vi "MOV_Query.vi"(0 "System no.":i32=1 min=1 max=4 step=1, 2 "Axes to query":string[](array[string]), 3 "All axes?":bool, 4 "Axis identifier?":bool=TRUE, 5 "error in":errorcluster) -> (14 "Target position":dbl[](array[numeric]) format="%.6f", 19 "error out":errorcluster)   [LabVIEW 2020]
doc: "GCS 3.0\n=====\n\nMOV? (Get Target Position) \n\nDescription \nQueries the currently valid target position for the axes.\n\nFormat\nMOV?[ <AxisID>]\n\nArguments\nMOV? without arguments queries all axes of the controller.\n<AxisID>\nAn axis of the controller\nThe response to USG? CMD MOV? indicates in the #Related Units block for which axes the \ncommand can be used.\nPossible values: Alias of the axis (p. 94) \n\nResponse\n<AxisID>\"=\"<TargetPosition> LF}\n<TargetPosition>\nCurrent target position in physical units\nThe data format is float.\nPossible values: Dependent on the permitted travel range of the axis\n\nExample\nIn this example, axis 2 does not support the mode of operation 0x2.\n>>MOV?\n<<AXIS_1=0.0\n<<AXIS_3=2.4\n>>MOV? AXIS_1\n<<AXIS_1=0.0\n\nNotes\nThe parameter Axis_n - 0x102 Target Position shows the current target position (in the physical \nunit of the axis). The value of this parameter can be read from the working memory of the \ncontroller using the SPV? command (p. 63); example for axis 1:\n>>spv? ram axis_1 - 0x102\n<<RAM AXIS_1 - 0x102=0.0\n\nUser command level\nUSR\n\n\nGCS 2.0\n=====\n\nReturns commanded target position.\n\nE-516: If All axes? = TRUE, then Axis identifier? must be TRUE\nE-710: If All axes? = TRUE, then Axis identifier? must be TRUE\nE-755: If All axes? = TRUE, then Axis identifier? can be FALSE. Command not available for E-755.101.\nE-816: All axes? = FALSE, only one axis per command allowed. \nF-206: For GCS syntax version = GCS 1.0 (check with CSV?.vi. If CSV?.vi is not supported, syntax version is GCS 1.0), cCommand has different implementation, please use MOV?_old.vi\nC-887, M-8X0: For GCS syntax version = GCS 1.0 (check with CSV?.vi. If CSV?.vi is not supported, syntax version is GCS 1.0), Ccommand has different implementation, please use MOV?_old.vi\nAll other systems: If All axes? = TRUE, then Axis identifier? can be FALSE"
panel:
  # "MOV? (Get Target Position) \n\nQueries the currently valid target position for the axes."
  # "Query"
  # "If all axes: use"
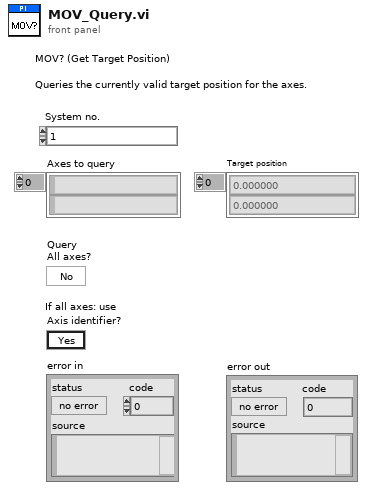
[diagram p1: front panel]
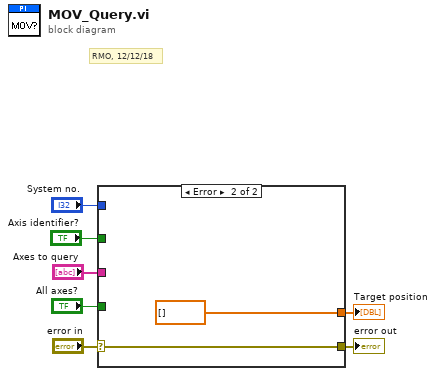
[diagram p0: block diagram]
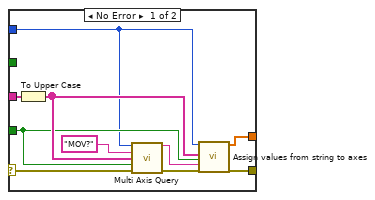
[diagram p2: hidden frame]
diagram:
  # "RMO, 12/12/18"
  n1 = case shown="Error" "error in" {
    selector: "error in" -> [w16 w19]
    tunnel: [w11 dbl[] [] ("Values")] -> w3
    tunnel: "Axes to query" -> [w17 _]
    tunnel: [w13 w19] -> w2
    tunnel: "System no." -> [w8 _]
    tunnel: "All axes?" -> [w9 _]
    tunnel: "Axis identifier?" -> [_ _]
    frame No Error {
      n2 = To Upper Case(1:w17) -> (0:w12:string[])
      n3 = call "Multi Axis Query.vi"("System no."=w8, "Command"="MOV?", "Axis"=w12, "All axes?"=w9, "error in (no error)"=w16) -> ("Answer"=w10:string, "error out"=w14:errorcluster)  [unwired: 9 in]
      n4 = call "Assign values from string to axes.vi"("System no."=w8, "Queried axes"=w12, "All axes queried?"=w9, "Input String"=w10, "error in"=w14) -> ("Values"=w11:dbl[], "error out"=w13:errorcluster)  [unwired: 4 in, 9 out]
    }
    frame Error {
      (unwired) string[] [] ("Axes to query out")
    }
  }
  "error out" <- w2
  "Target position" <- w3
